vi "3_1.vi"() -> ()   [LabVIEW 2010]
uses:
  Control 1.ctl
panel:
  out "Таблиця 1 - Вхідні дані 2":string[][](table)
  in  "Таблиця 1 - Вхідні дані":string[][](table)
  in  "4":bool
  in  "3":bool
  in  "2":bool
  in  "1":bool
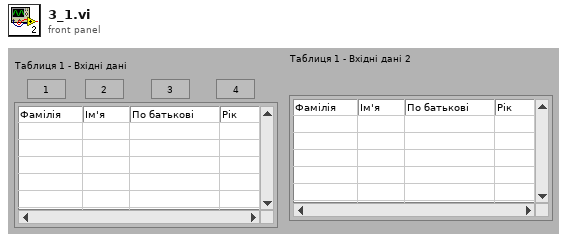
[diagram p1: front panel]
types:
  T1 = typedef "Control 1.ctl" = enum16{"Стоп", "1", "2", "3", "4"}
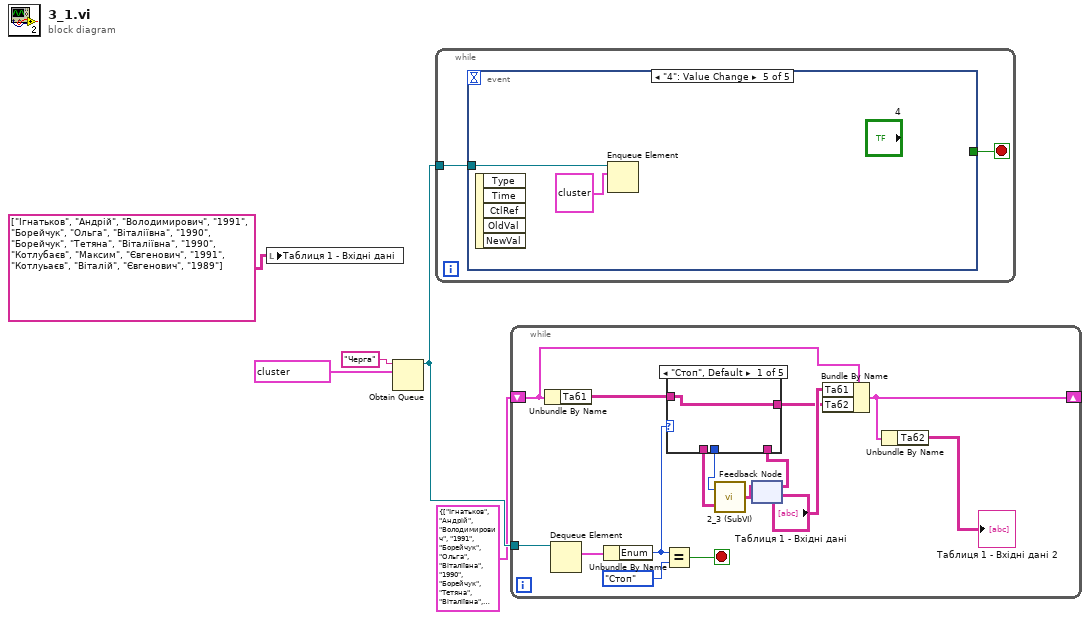
[diagram p0: block diagram]
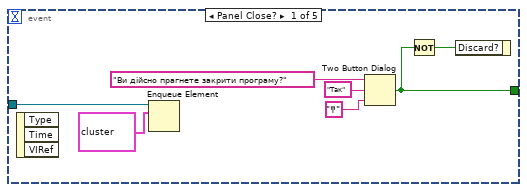
[diagram p2: hidden frame]
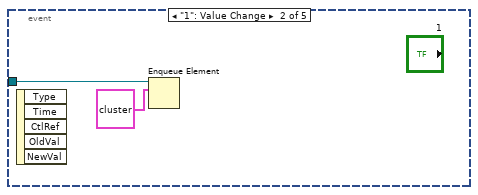
[diagram p3: hidden frame]
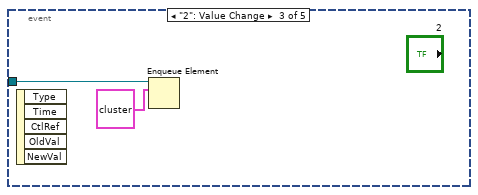
[diagram p4: hidden frame]
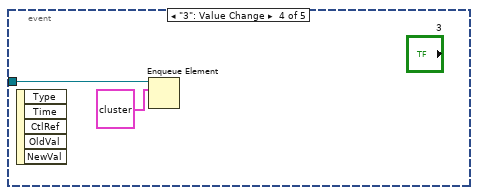
[diagram p5: hidden frame]
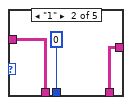
[diagram p6: hidden frame]
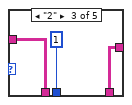
[diagram p7: hidden frame]
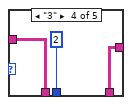
[diagram p8: hidden frame]
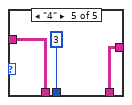
[diagram p9: hidden frame]
diagram:
  n1 = local write "Таблиця 1 - Вхідні дані"(string[][] [["Ігнатьков", "Андрій", "Володимирович", "1991"], ["Борейчук", "Ольга", "Віталіївна", "1990"], ["Борейчук", "Тетяна", "Віталіївна", "1990"], ["Котлубаєв", "Максим", "Євгенович", "1991"], ["Котлуьаєв", "Віталій", "Євгенович", "1989"]] ("Таблиця 1")) -> ()
  n2 = Obtain Queue(name (unnamed)="Черга", element data type=cluster{"variant":variant, "Enum":T1} {"variant"=variant, "Enum"=enum."Стоп"}) -> (queue out=w3:refnum<queue>)  [unwired: 3 in, 2 out]
  n3 = while {
    tunnel: w3 -> [w6]
    stop <- w7 stop-if-true
    n4 = event shown="[4] \"4\": Value Change" {
      selector: _ -> [_ _ _ _ _]
      dyn-events: _ -> [_ _ _ _ _]
      timeout: _ -> [_ _ _ _ _]
      tunnel: [w10 _ _ _ _] -> w7
      tunnel: w6 -> [w9 w15 w17 w19 w21]
      event Panel Close? {
        n5 = event-data() -> ()  [unwired: 1 in, 3 out]
        n6 = Enqueue Element(queue=w9, element=cluster{"variant":variant, "Enum":T1} {"variant"=variant, "Enum"=enum."Стоп"}) -> ()  [unwired: 2 in, 3 out]
        n7 = Two Button Dialog(message="Ви дійсно прагнете закрити програму?", 1:"ͳ" ("F button name (\"Cancel\")"), 2:"Так" ("T button name (\"OK\")")) -> (T button?=w10:bool)
        n8 = Not(x=w10) -> (.not. x?=w11:bool)
        n9 = event-data("Discard?"=w11) -> ()  [unwired: 1 in, 1 out]
      }
      event "1": Value Change {
        n10 = event-data() -> ()  [unwired: 1 in, 5 out]
        n11 = Enqueue Element(queue=w15, element=cluster{"variant":variant, "Enum":T1} {"variant"=variant, "Enum"=enum."1"}) -> ()  [unwired: 2 in, 3 out]
      }
      event "2": Value Change {
        n12 = event-data() -> ()  [unwired: 1 in, 5 out]
        n13 = Enqueue Element(queue=w17, element=cluster{"variant":variant, "Enum":T1} {"variant"=variant, "Enum"=enum."2"}) -> ()  [unwired: 2 in, 3 out]
      }
      event "3": Value Change {
        n14 = event-data() -> ()  [unwired: 1 in, 5 out]
        n15 = Enqueue Element(queue=w19, element=cluster{"variant":variant, "Enum":T1} {"variant"=variant, "Enum"=enum."3"}) -> ()  [unwired: 2 in, 3 out]
      }
      event "4": Value Change {
        n16 = event-data() -> ()  [unwired: 1 in, 5 out]
        n17 = Enqueue Element(queue=w21, element=cluster{"variant":variant, "Enum":T1} {"variant"=variant, "Enum"=enum."3"}) -> ()  [unwired: 2 in, 3 out]
      }
    }
  }
  n18 = while {
    tunnel: w3 -> [w37]
    shift-right: [w28] -> _
    shift-left: cluster{"Таб1":string[][], "Таб2":string[][]} {"Таб1"=[["Ігнатьков", "Андрій", "Володимирович", "1991"], ["Борейчук", "Ольга", "Віталіївна", "1990"], ["Борейчук", "Тетяна", "Віталіївна", "1990"], ["Котлубаєв", "Максим", "Євгенович", "1991"], ["Котлуьаєв", "Віталій", "Євгенович", "1989"]], "Таб2"=[["Ігнатьков", "Андрій", "Володимирович", "1991"], ["Борейчук", "Ольга", "Віталіївна", "1990"], ["Борейчук", "Тетяна", "Віталіївна", "1990"], ["Котлубаєв", "Максим", "Євгенович", "1991"], ["Котлуьаєв", "Віталій", "Євгенович", "1989"]]} -> [w30]
    stop <- w34 stop-if-true
    n19 = Unbundle By Name(w30) -> ("Таб1"=w32:string[][])
    n20 = Dequeue Element(queue=w37) -> (element=w36:cluster{"variant":variant, "Enum":T1})  [unwired: 2 in, 3 out]
    n21 = Unbundle By Name(w36) -> ("Enum"=w33:T1)
    n22 = Equal?(x=w33, y=Control_1."Стоп" ("Enum")) -> (x = y?=w34:bool)
    n23 = feedback #1() -> (w24:string[][])  [unwired: 1 in]
    n24 = case shown="\"Стоп\", Default" w33 {
      tunnel: w32 -> [w38 w41 w44 w46 w50]
      tunnel: [w38 w40 w42 w47 w49] -> w29
      tunnel: [_ w41 w44 w46 w50] -> w26
      tunnel: w24 -> [_ w40 w42 w47 w49]
      tunnel: [_ 0 ("Сортувати стовпчик") 1 ("Сортувати стовпчик") 2 ("Сортувати стовпчик") 3 ("Сортувати стовпчик")] -> w23
      frame "Стоп", Default {
      }
      frame "1" {
      }
      frame "2" {
      }
      frame "3" {
      }
      frame "4" {
      }
    }
    n25 = call "2_3 (SubVI).vi"("Таблиця 1 - Вхідні дані"=w26, "Сортувати стовпчик"=w23) -> ("Таблиця 2 - Результат"=w25:string[][])
    n26 = feedback-in #1(w25) -> ()
    n27 = Bundle By Name(cluster=w30, "Таб1"="Таблиця 1 - Вхідні дані", "Таб2"=w29) -> (w28:cluster{"Таб1":string[][], "Таб2":string[][]})
    n28 = Unbundle By Name(w28) -> ("Таб2"=→"Таблиця 1 - Вхідні дані 2":string[][])
  }
